vi "Do.vi"(8 "error in (no error)":errorcluster, 10 "Actor in":refnum<class "Actor.lvclass">, 11 "Multiplication Task Msg":refnum<class "Multiplication Task Msg.lvclass">) -> (0 "error out":errorcluster, 2 "Actor out":refnum<class "Actor.lvclass">)   [LabVIEW 2015, in "Multiplication Actor.lvlib" / "Multiplication Task Msg.lvclass"]
uses:
  Multiplication Task Msg.lvclass
  <vilib>/ActorFramework/Actor/Actor.lvclass
  Multiplication/Multiplication.lvclass
  Multiplication Task Msg.lvclass/Multiplication Task Msg.ctl
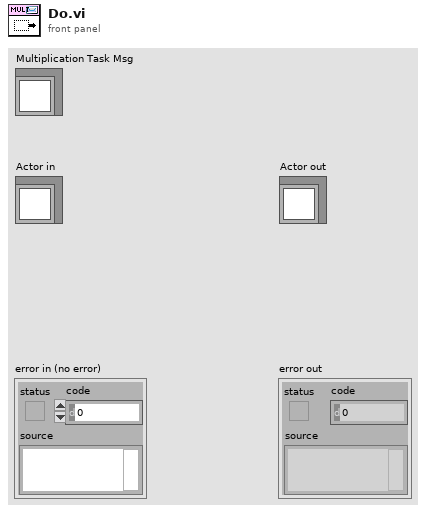
[diagram p1: front panel]
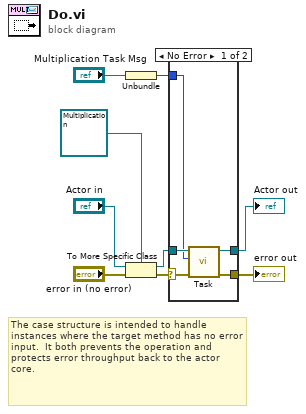
[diagram p0: block diagram]
diagram:
  # "The case structure is intended to handle instances where the target method has no error input.  It both prevents the operation and protects error throughput back to the actor core."
  n1 = Unbundle("Multiplication Task Msg") -> (w1:i32)
  n2 = To More Specific Class(target class=refnum<class "Multiplication.lvclass"> refnum ("Actor in"), reference="Actor in", error in="error in (no error)") -> (specific class reference=w8:refnum<class "Multiplication.lvclass">, error out=w4:errorcluster)
  n3 = case shown="No Error" w4 {
    selector: w4 -> [w11 w16]
    tunnel: w8 -> [w14 w15]
    tunnel: [w13 w16] -> w3
    tunnel: [w12 w15] -> w2
    tunnel: w1 -> [w10 _]
    frame No Error {
      n4 = call-dynamic "Task.vi"("error in (no error)"=w11, "Data"=w10, "Multiplication in"=w14) -> ("error out"=w13:errorcluster, "Multiplication out"=w12:refnum<class "Multiplication.lvclass">)  [unwired: 7 in]
    }
    frame Error {
    }
  }
  "error out" <- w3
  "Actor out" <- w2
